vi "List Queues.vi"(6 "Name Prefix":string, 8 "error in (no error)":errorcluster, 9 "Region":T1, 11 "AWS Credentials":T2) -> (0 "error out":errorcluster, 3 "SQS Queues":refnum<class "NI_AWS_SQS.lvclass">[](array[class]))   [LabVIEW 2015, in "NI_AWS_SQS.lvclass"]
uses:
  NI_AWS_SQS.lvclass
  Core/AWS Credentials.ctl
  Core/Region.ctl
  Core/Request Options.ctl
  Core/Name Value Pair.ctl
  Core/NI_AWS_Core.lvclass/NI_AWS_Core.ctl
  NI_AWS_SQS.lvclass/NI_AWS_SQS.ctl
  Write Account Number.vi
  Write Name.vi
  Write URL.vi
  Core/Write Credentials.vi
  Core/Write Region.vi
  Core/Write Service.vi
  Core/Write Verify Server.vi
  Core/NI_AWS_Core.lvclass
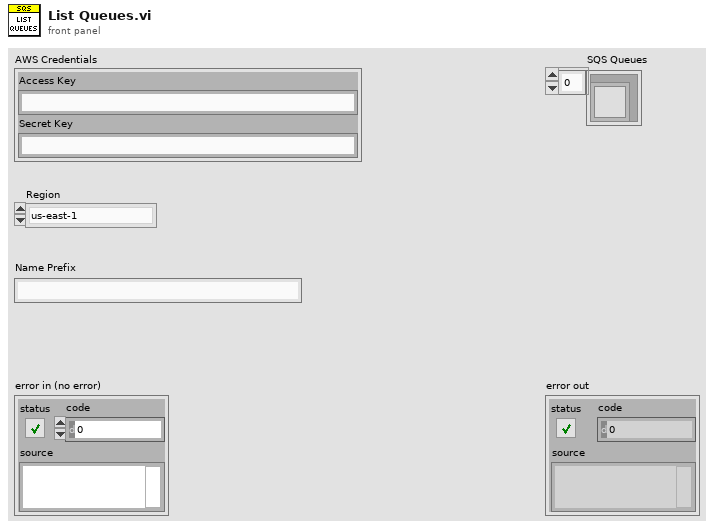
[diagram p1: front panel]
types:
  T1 = typedef "NI_AWS_Core.lvclass/Region.ctl" = enum16{"us-east-1", "us-east-2", "us-west-1", "us-west-2", "ap-northeast-1", "ap-northeast-2", "ap-southeast-1", "ap-southeast-2", "ca-central-1", "eu-central-1", "eu-west-1", "eu-west-2", "sa-east-1"}
  T2 = typedef "NI_AWS_Core.lvclass/AWS Credentials.ctl" = cluster{"Access Key":string, "Secret Key":string}
  T3 = typedef "NI_AWS_Core.lvclass/Name Value Pair.ctl" = cluster{"name":string, "value":string}
  T4 = typedef "NI_AWS_Core.lvclass/Request Options.ctl" = cluster{"request headers":T3[], "request parameters":T3[], "request body":string}
  T5 = typedef "NI_AWS_Core.lvclass/Response.ctl" = cluster{"Headers":string, "Body":string}
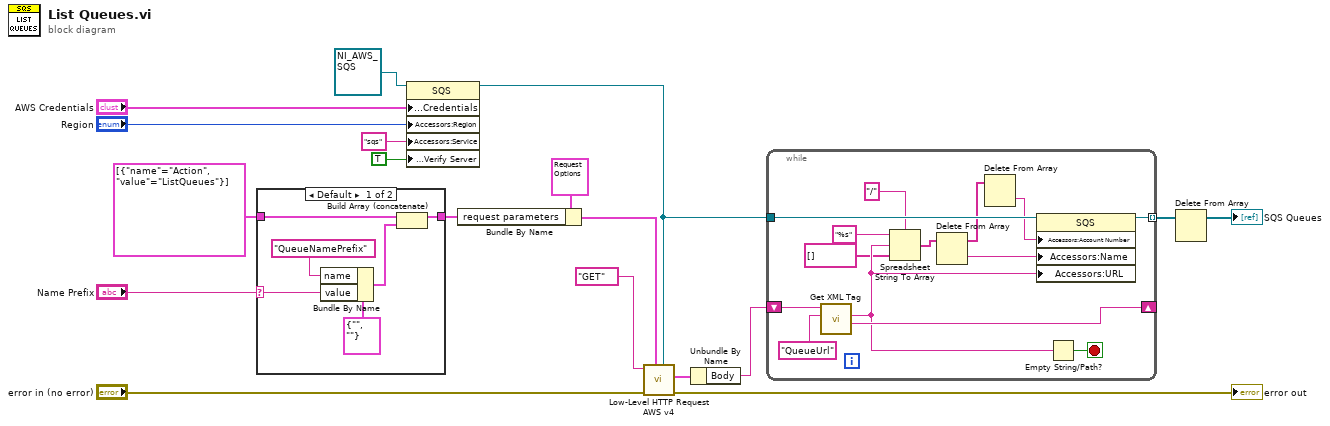
[diagram p0: block diagram]
diagram:
  n1 = case shown="Default" "Name Prefix" {
    selector: "Name Prefix" -> [w20 _]
    tunnel: T3[] [{"name"="Action", "value"="ListQueues"}] ("request parameters") -> [w24 w25]
    tunnel: [w23 w25] -> w8
    frame Default {
      n2 = Bundle By Name(cluster=T3 {"name"="", "value"=""} ("Cluster"), "name"="QueueNamePrefix", "value"=w20) -> (w21:T3)
      n3 = Build Array (concatenate)(w24, w21) -> (w23:T3[])
    }
    frame "" {
    }
  }
  n4 = property class="SQS"(reference=refnum<class "NI_AWS_SQS.lvclass"> refnum ("NI_SQS.lvlib:SQS"), "Accessors:Credentials"="AWS Credentials", "Accessors:Region"="Region", "Accessors:Service"="sqs" ("Service"), "Accessors:Verify Server"=TRUE ("Verify Server")) -> (reference out=w3:refnum<class "NI_AWS_SQS.lvclass">)  [unwired: 1 in, 1 out]
  n5 = Bundle By Name(cluster=T4 {"request headers"=[], "request parameters"=[{"name"="Action", "value"="ListQueues"}], "request body"=""} ("Request Options"), "request parameters"=w8) -> (w10:T4)
  n6 = call "Low-Level HTTP Request AWS v4.vi"("AWS Core"=w3, "Request Options"=w10, "error in (no error)"="error in (no error)", "HTTP-Verb"="GET") -> ("error out"=→"error out":errorcluster, "Response"=w5:T5)  [unwired: 5 in, 1 out]
  n7 = Unbundle By Name(w5) -> ("Body"=w4:string)
  n8 = while {
    shift-right: [w38] -> _
    shift-left: w4 -> [w39]
    tunnel: w3 -> [w35]
    tunnel: [w34] -> w2 mode=indexing
    stop <- w37 stop-if-true
    n9 = call "Get XML Tag.vi"("Tag name"="QueueUrl", "XML String in"=w39) -> ("Remaining string"=w38:string, "Tag value"=w33:string)  [unwired: 5 in, 3 out]
    n10 = Spreadsheet String To Array(delimiter (Tab)="/", format string="%s", spreadsheet string=w33, array type (2D Dbl)=string[] []) -> (array=w29:string[])
    n11 = Delete From Array(array=w29) -> (deleted portion=w28:string, array with subset deleted=w27:string[])  [unwired: 2 in]
    n12 = Delete From Array(array=w27) -> (deleted portion=w26:string)  [unwired: 2 in, 1 out]
    n13 = property class="SQS"(reference=w35, "Accessors:Account Number"=w26, "Accessors:Name"=w28, "Accessors:URL"=w33) -> (reference out=w34:refnum<class "NI_AWS_SQS.lvclass">)  [unwired: 1 in, 1 out]
    n14 = Empty String/Path?(string/path=w33) -> (empty?=w37:bool)
  }
  n15 = Delete From Array(array=w2) -> (array with subset deleted=→"SQS Queues":refnum<class "NI_AWS_SQS.lvclass">[])  [unwired: 2 in, 1 out]
